vi "TryUpdateInclinometerError.vi"   [LabVIEW 2016]
uses:
  TelemetryDataTypes.ctl
  TelemetryUpdateModes.ctl
  TelemetryFields.ctl
  <vilib>/rvi/Emulation/niFpgaEmulationIsFPGAContextNoSignature.vi
  <vilib>/rvi/Emulation/niFpgaSctlEmulationGetInTimedLoop.vi
  <vilib>/rvi/errors/niFpgaSetErrorForExecOnDevCompSimple.vi
  <vilib>/rvi/eio/common/nirviEmuReportErrorAndStop.vi
  <vilib>/rvi/DataTransferAndStorage/Container/Common/niFpgaContainerGetUniqueNameForEmu.vi
  <vilib>/rvi/FIFO/Fifo_Resource/nirvififoEmulationSetSize.vi
  <vilib>/rvi/FIFO/Fifo_Resource/nirviFifoEmulationQueueMgr.vi
  <instcachedir>/0/nirviFifoEmulationQueueMgr_E5CAEC123FF24DC58D834DCA3CDAA9B5.lvgen/nirviFifoEmulationQueueMgr_E5CAEC123FF24DC58D834DCA3CDAA9B5_033.vi
  <vilib>/Utility/error.llb/Clear Errors.vi
  <vilib>/rvi/FIFO/Fifo_Resource/nirvififoEmulationCreateLock.vi
  <vilib>/rvi/Emulation/niFpgaProcessEmulError.vi
  <vilib>/rvi/FIFO/Fifo_Resource/nirvififoEmulationObtainLock.vi
  <vilib>/rvi/FIFO/Fifo_Resource/nirvififoEmulationReleaseLock.vi
  <vilib>/rvi/occurrence/nirviWaitOnOccurrenceBase.vi
  <vilib>/rvi/errors/nirviReportUnexpectedCaseInternalError.vi
  <vilib>/rvi/errors/nirviReportUnexpectedCaseInternalError (U32).vi
  <instcachedir>/0/nirviFifoEmulationQueueMgr_E5CAEC123FF24DC58D834DCA3CDAA9B5.lvgen/nirviFifoEmulationQueueMgr_E5CAEC123FF24DC58D834DCA3CDAA9B5_030.vi
  <vilib>/rvi/FIFO/Fifo_Resource/nirvififoEmulationDetermineInputValidOut.vi
  <vilib>/rvi/Emulation/niFpgaGetClockAttributes.vi
  <vilib>/rvi/Emulation/niFpgaEmulationReportErrorSimple.vi
  <vilib>/rvi/Emulation/niFpgaCriticalErrorInLSC.vi
  <vilib>/rvi/DataTransferAndStorage/Container/XNode/niFpgaContainer.xnode
  <vilib>/rvi/FIFO/Fifo_Resource/nirvififoEmulationRead.vi
  <vilib>/rvi/FIFO/Fifo_Resource/nirvififoEmulationWrite.vi
  <vilib>/rvi/FIFO/Fifo_Resource/nirvififoEmulationGetNumberOfElementsToRead.vi
types:
  T1 = cluster{"Timestamp":u64, "TxBytes":u64, "RxBytes":u64, "TxFrames":u64, "RxFrames":u64, "ErrorCode":enum8{"None", "ResponseAddressError", "ResponseFunctionCodeError", "ResponseByteCountError", "ResponseCRCError", "ResponseUnknownError", "ResponseTimeoutError", "SensorReportsIllegalFunction", "SensorReportsIllegalDataAddress"}}
  T2 = typedef "TelemetryFields.ctl" = enum16{"None", "InclinometerTxBytes", "InclinometerRxBytes", "InclinometerTxFrames", "InclinometerRxFrames", "InclinometerErrorTimestamp", "InclinometerErrorCode", "InclinometerSampleTimestamp", "InclinometerRawAngle", "InclinometerZenithAngle", "DisplacementTxBytes", "DisplacementRxBytes", "DisplacementTxFrames", "DisplacementRxFrames", "DisplacementErrorTimestamp", "DisplacementErrorCode", "DisplacementSampleTimestamp", "DisplacementRaw1", "DisplacementRaw2", "DisplacementRaw3", "DisplacementRaw4", "DisplacementRaw5", "DisplacementRaw6", "DisplacementRaw7", "DisplacementRaw8", "DisplacementEng1", "DisplacementEng2", "DisplacementEng3", "DisplacementEng4", "DisplacementEng5", "DisplacementEng6", "DisplacementEng7", "DisplacementEng8", "DisplacementPositionX", "DisplacementPositionY", "DisplacementPositionZ", "DisplacementRotationX", "DisplacementRotationY", "DisplacementRotationZ", "AccelerometerSampleCount", "AccelerometerTimestamp", "AccelerometerRaw1", "AccelerometerRaw2", "AccelerometerRaw3", "AccelerometerRaw4", "AccelerometerRaw5", "AccelerometerRaw6", "AccelerometerRaw7", "AccelerometerRaw8", "AccelerometerEng1", "AccelerometerEng2", "AccelerometerEng3", "AccelerometerEng4", "AccelerometerEng5", "AccelerometerEng6", "AccelerometerEng7", "AccelerometerEng8", "AngularAccelerationX", "AngularAccelerationY", "AngularAccelerationZ"}
  T3 = typedef "TelemetryUpdateModes.ctl" = enum8{"=", "+", "-", "|"}
  T4 = typedef "TelemetryDataTypes.ctl" = enum8{"U8", "U16", "U32", "U64", "I8", "I16", "I32", "I64", "SGL"}
  T5 = typedef "TelemetryUpdateData.ctl" = cluster{"DataType":T4, "Mode":T3, "Field":T2, "Data":u64}
  T6 = enum8{"None", "ResponseAddressError", "ResponseFunctionCodeError", "ResponseByteCountError", "ResponseCRCError", "ResponseUnknownError", "ResponseTimeoutError", "SensorReportsIllegalFunction", "SensorReportsIllegalDataAddress"}
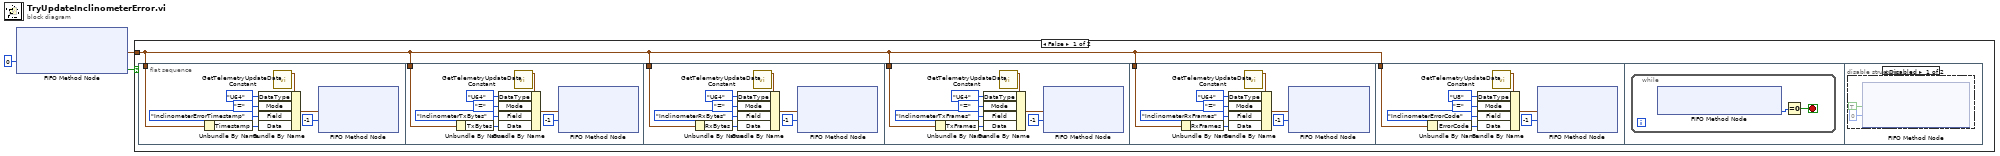
[diagram p0: block diagram]
diagram:
  n1 = xnode ("FIFO Method Node")("Timeout"=0) -> ("Element"=w1:T1, "Timed Out?"=w2:bool)  [unwired: 1 in, 1 out]
  n2 = case shown="False" w2 {
    tunnel: w1 -> [w4 _]
    frame False {
      n3 = flat-sequence {
        tunnel: w4 -> [w7]
        tunnel: w4 -> [w13]
        tunnel: w4 -> [w21]
        tunnel: w4 -> [w29]
        tunnel: w4 -> [w37]
        tunnel: w4 -> [w46]
        frame #0 {
          n4 = Unbundle By Name(w7) -> ("Timestamp"=w6:u64)
          n5 = call "GetTelemetryUpdateDataConstant.vi"() -> ("TelemetryUpdateData"=w8:T5)  [unwired: 11 in]
          n6 = Bundle By Name(cluster=w8, "DataType"=TelemetryDataTypes."U64", "Mode"=TelemetryUpdateModes."=", "Field"=TelemetryFields."InclinometerErrorTimestamp" ("TelemetryFields"), "Data"=w6) -> (w11:T5)
          n7 = xnode ("FIFO Method Node")("Element"=w11, "Timeout"=-1) -> ()  [unwired: 1 in, 2 out]
        }
        frame #1 {
          n8 = Unbundle By Name(w13) -> ("TxBytes"=w20:u64)
          n9 = call "GetTelemetryUpdateDataConstant.vi"() -> ("TelemetryUpdateData"=w19:T5)  [unwired: 11 in]
          n10 = Bundle By Name(cluster=w19, "DataType"=TelemetryDataTypes."U64", "Mode"=TelemetryUpdateModes."=", "Field"=TelemetryFields."InclinometerTxBytes", "Data"=w20) -> (w15:T5)
          n11 = xnode ("FIFO Method Node")("Element"=w15, "Timeout"=-1) -> ()  [unwired: 1 in, 2 out]
        }
        frame #2 {
          n12 = Unbundle By Name(w21) -> ("RxBytes"=w22:u64)
          n13 = call "GetTelemetryUpdateDataConstant.vi"() -> ("TelemetryUpdateData"=w23:T5)  [unwired: 11 in]
          n14 = Bundle By Name(cluster=w23, "DataType"=TelemetryDataTypes."U64", "Mode"=TelemetryUpdateModes."=", "Field"=TelemetryFields."InclinometerRxBytes", "Data"=w22) -> (w27:T5)
          n15 = xnode ("FIFO Method Node")("Element"=w27, "Timeout"=-1) -> ()  [unwired: 1 in, 2 out]
        }
        frame #3 {
          n16 = Unbundle By Name(w29) -> ("TxFrames"=w36:u64)
          n17 = call "GetTelemetryUpdateDataConstant.vi"() -> ("TelemetryUpdateData"=w35:T5)  [unwired: 11 in]
          n18 = Bundle By Name(cluster=w35, "DataType"=TelemetryDataTypes."U64", "Mode"=TelemetryUpdateModes."=", "Field"=TelemetryFields."InclinometerTxFrames", "Data"=w36) -> (w31:T5)
          n19 = xnode ("FIFO Method Node")("Element"=w31, "Timeout"=-1) -> ()  [unwired: 1 in, 2 out]
        }
        frame #4 {
          n20 = Unbundle By Name(w37) -> ("RxFrames"=w38:u64)
          n21 = call "GetTelemetryUpdateDataConstant.vi"() -> ("TelemetryUpdateData"=w39:T5)  [unwired: 11 in]
          n22 = Bundle By Name(cluster=w39, "DataType"=TelemetryDataTypes."U64", "Mode"=TelemetryUpdateModes."=", "Field"=TelemetryFields."InclinometerRxFrames", "Data"=w38) -> (w43:T5)
          n23 = xnode ("FIFO Method Node")("Element"=w43, "Timeout"=-1) -> ()  [unwired: 1 in, 2 out]
        }
        frame #5 {
          n24 = Unbundle By Name(w46) -> ("ErrorCode"=w52:T6)
          n25 = call "GetTelemetryUpdateDataConstant.vi"() -> ("TelemetryUpdateData"=w51:T5)  [unwired: 11 in]
          n26 = Bundle By Name(cluster=w51, "DataType"=TelemetryDataTypes."U8", "Mode"=TelemetryUpdateModes."=", "Field"=TelemetryFields."InclinometerErrorCode" ("TelemetryFields"), "Data"=w52) -> (w48:T5)
          n27 = xnode ("FIFO Method Node")("Element"=w48, "Timeout"=-1) -> ()  [unwired: 1 in, 2 out]
        }
        frame #6 {
          n28 = while {
            stop <- w53 stop-if-true
            n29 = xnode ("FIFO Method Node")() -> ("Number of Elements to Read"=w54:u32)  [unwired: 1 in, 1 out]
            n30 = Equal To 0?(x=w54) -> (x = 0?=w53:bool)
          }
        }
        frame #7 {
          n31 = disable-structure shown="Disabled" {
            frame Disabled {
              n32 = xnode ("FIFO Method Node")("Element"=TRUE, "Timeout"=0) -> ()  [unwired: 1 in, 2 out]
            }
            frame Enabled {
            }
          }
        }
      }
    }
    frame True {
    }
  }
